vi "PH_Cont-601k_PSU.evt Call Set Flash Interval.vi"(0 "i ref in":refnum<vi>, 1 "Instance name":string="N/A", 4 "Flash Interval [s]":dbl, 5 "error in":errorcluster) -> (14 "i ref out":refnum<vi>, 19 "error out":errorcluster)   [LabVIEW 2014, in "PH_Cont-601k_PSU.lvlib"]
doc: "This VI calls an event by a simple call."
uses:
  PH_Cont-601k_PSU.lvlib
  CS_Core/CSSystem/CoreLib/CoreLib.double 2 byte array.vi
  CS_Core/BaseProcess/BaseProcess.lvlib
  CS_Core/CSSystem/CoreLib/CoreLib.lvlib
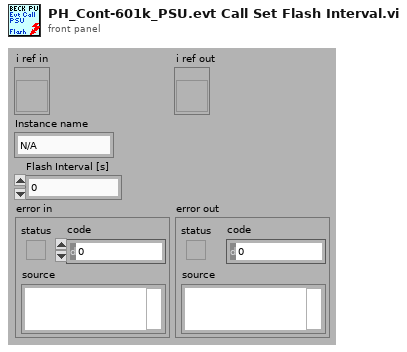
[diagram p1: front panel]
types:
  T1 = typedef "CoreDefs.rawDataType.ctl" = i8[]
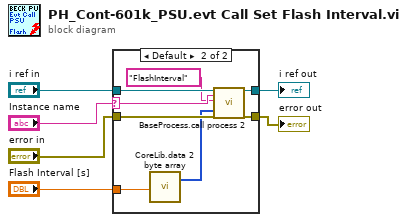
[diagram p0: block diagram]
diagram:
  n1 = case shown="Default" "Instance name" {
    selector: "Instance name" -> [_ w12]
    tunnel: [w7 w16] -> w6
    tunnel: "error in" -> [w7 w15]
    tunnel: [w8 w14] -> w3
    tunnel: "i ref in" -> [w8 w13]
    tunnel: "Flash Interval [s]" -> [_ w9]
    frame "", "N/A" {
    }
    frame Default {
      n2 = call-poly "CoreLib.data 2 byte array.vi"("f64"=w9) -> ("byteArray out"=w10:T1)  [unwired: 18 in]
      n3 = call "BaseProcess.call process 2.vi"("i ref in"=w13, "Object"=w12, "Selector"="FlashInterval", "Data"=w10, "error in (no error)"=w15) -> ("i ref out"=w14:refnum<vi>, "error out"=w16:errorcluster)  [unwired: 13 in]
    }
  }
  "error out" <- w6
  "i ref out" <- w3
